vi "Example_Easy Save or Load Controls To From File.vi"() -> ()   [LabVIEW 2020]
doc: "Demonstrates how GUI object values can be saved into configuration file or loaded from the configuration file. This feature is extremely useful to manage settings of the application. Another, and very important, feature is that adding or removing items to be saved is taking minimum time."
uses:
  VI Server Toolkit LV2013.lvlib
  VI Server Libraries/VI Server Controls.llb/VI Server_GetSet Controls From String Format_Options.ctl
panel:
  in  "2D Array - Boolean":bool[][](array[boolean]) caption="2D Array - String"
  in  "2D Array - Path":path[][](array[path]) caption="2D Array - String"
  in  "EXIT":bool
  in  "LED":bool
  in  "Error In":errorcluster
  out "error out":errorcluster
  in  "SystemConfigurationFile":path caption="System Configuration File"
  in  "Load":bool
  in  "Save":bool
  in  "2D Array - String":string[][](array[string])
  in  "2D Array - DBL":dbl[][](array[numeric])
  in  "Menu Ring":u16(ring) items=["Item 1", "Item 2", "Item 3"]
  in  "1D Array - DBL":dbl[](array[numeric])
  in  "1D Array - String":string[](array[string])
  in  "Settings Button":bool
  in  "Knob":dbl(knob)=0.15380597915361302 scale=0.0..10.0
  in  "Horizontal Fill Slide":dbl(slide) scale=0.0..10.0
  in  "Numeric Control":dbl
  # "INSTRUCTIONS:\n\n1. Create the \"System configuration\" file path.\n2. Populate array elements, set controls and ring selection.\n3. Save the settings into configuration file (SAVE button).\n4. Change settings, empty arrays.\n5. Press LOAD button and verify the settings are properly updated.\n6. Examine the block diagram and note the Control Labels array which contains \nall labels of the saved/loaded controls."
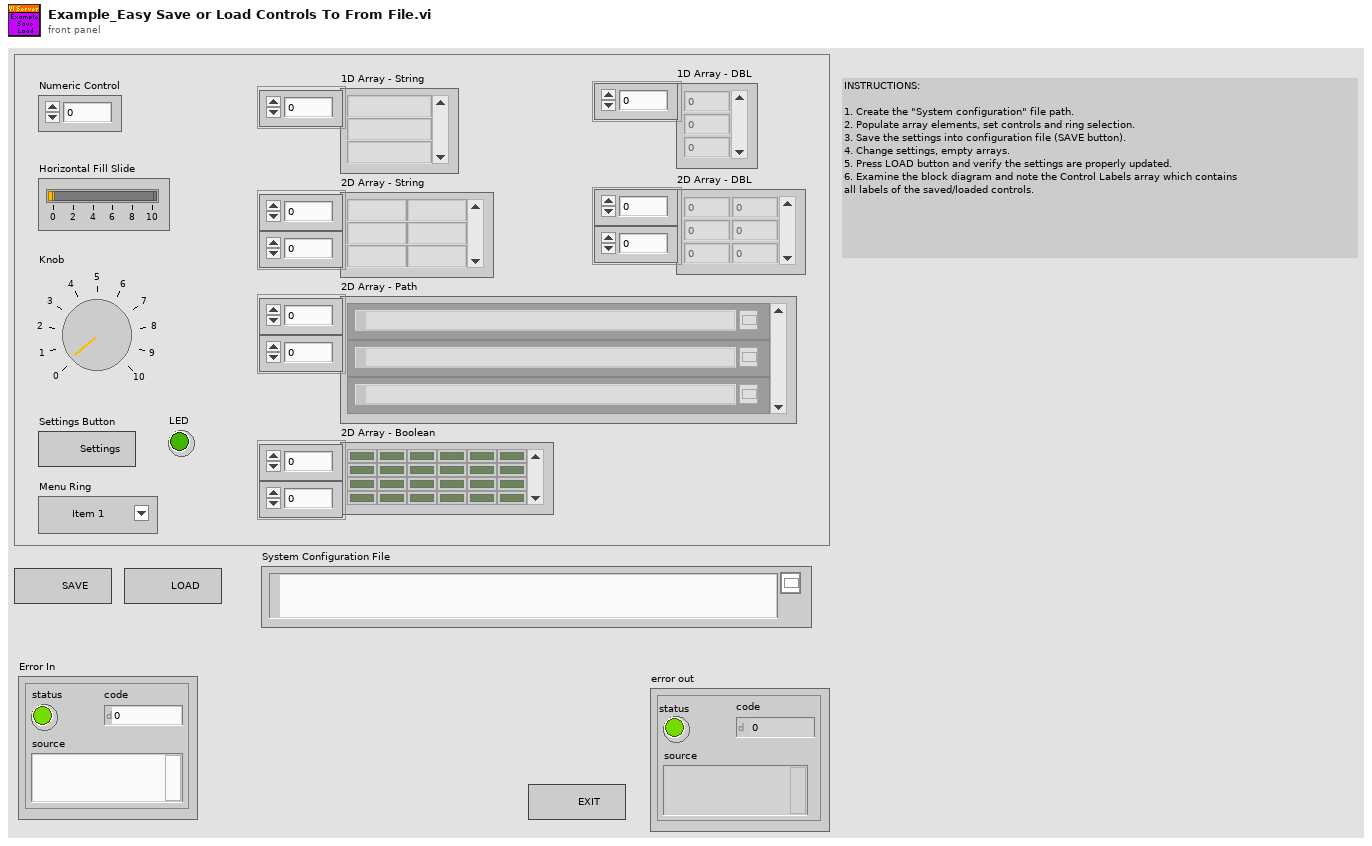
[diagram p1: front panel]
types:
  T1 = typedef "VI Server_RefsCluster.ctl" = cluster{"Labels":string[], "Refs":refnum<vi>[], "VI Ref":refnum<vi>}
  T2 = typedef "VI Server Toolkit LV2013.lvlib/VI Server_GetSet Controls From String Format_Options.ctl" = enum16{"", "If Ring Get Selection", "If Ring Set by Selection"}
  T3 = enum8{"Enabled", "Disabled", "Disabled and Grayed Out"}[]
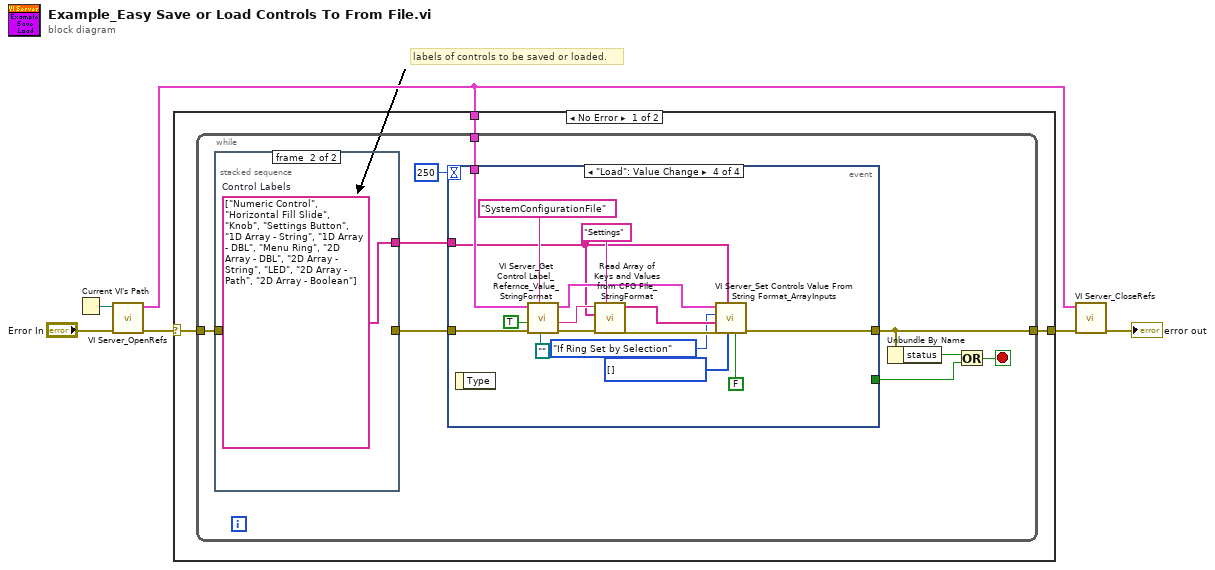
[diagram p0: block diagram]
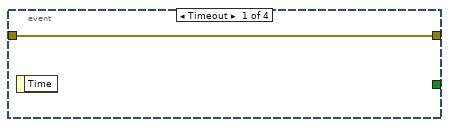
[diagram p2: hidden frame]
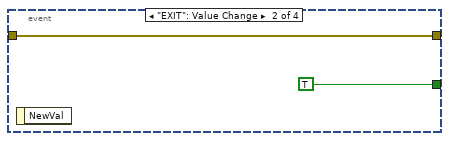
[diagram p3: hidden frame]
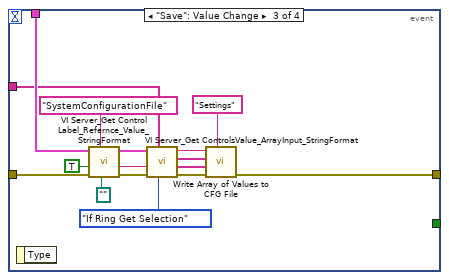
[diagram p4: hidden frame]
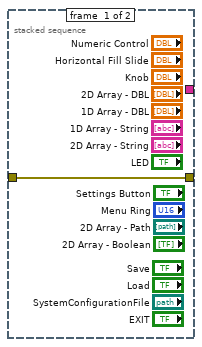
[diagram p5: hidden frame]
diagram:
  # "labels of controls to be saved or loaded."
  n1 = Current VI's Path() -> (path=w5:path)
  n2 = call "VI Server_OpenRefs.vi"("error in"="Error In", "VI Path"=w5) -> ("error out"=w4:errorcluster, "VI Server.RefsCluster"=w1:T1)  [unwired: 8 in]
  n3 = case shown="No Error" w4 {
    selector: w4 -> [w9 w55]
    tunnel: [w8 w55] -> w3
    tunnel: w1 -> [w7 _]
    frame No Error {
      n4 = while {
        tunnel: w9 -> [w17]
        tunnel: [w15] -> w8
        tunnel: w7 -> [w11]
        stop <- w12 stop-if-true
        n5 = stacked-sequence {
          tunnel: [w53 _] -> w16
          tunnel: w17 -> [w53 _]
          tunnel: [_ w54] -> w10
          frame #0 {
          }
          frame #1 {
            w54 = string[] ["Numeric Control", "Horizontal Fill Slide", "Knob", "Settings Button", "1D Array - String", "1D Array - DBL", "Menu Ring", "2D Array - DBL", "2D Array - String", "LED", "2D Array - Path", "2D Array - Boolean"]  # Control Labels
          }
        }
        n6 = event shown="[3] \"Load\": Value Change" {
          selector: _ -> [_ _ _ _]
          dyn-events: _ -> [_ _ _ _]
          timeout: 250 -> [_ _ _ _]
          tunnel: w16 -> [w19 w21 w33 w49]
          tunnel: [w19 w21 w22 w39] -> w15
          tunnel: [_ TRUE _ _] -> w13
          tunnel: w11 -> [_ _ w32 w48]
          tunnel: w10 -> [_ _ w28 w41]
          event Timeout {
            n7 = event-data() -> ()  [unwired: 1 in, 1 out]
          }
          event "EXIT": Value Change {
            n8 = event-data() -> ()  [unwired: 1 in, 1 out]
          }
          event "Save": Value Change {
            n9 = event-data() -> ()  [unwired: 1 in, 1 out]
            n10 = call "VI Server_Get Control Label_Refernce_Value_StringFormat.vi"(6:path "", "Label"="SystemConfigurationFile", "error in (no error)"=w33, 9:TRUE ("Single Instance (T)"), "VI Server Cluster"=w32) -> ("error out"=w31:errorcluster, "ControlValue(StringFormat)"=w26:string, "VI Server Cluster.DUP"=w30:T1)  [unwired: 4 in]
            n11 = call "VI Server_Get ControlsValue_ArrayInput_StringFormat.vi"("Options"=VI_Server_GetSet_Controls_From_String_Format_Options."If Ring Get Selection", "Labels.Array"=w28, "error in (no error)"=w31, "VI Server Cluster"=w30) -> ("error out"=w27:errorcluster, "Values.Array.STR"=w23:string[], "Labels.Array.DUP"=w24:string[])  [unwired: 3 in, 2 out]
            n12 = call "Write Array of Values to CFG File.vi"("Section"="Settings", "error in"=w27, "ValuesArray"=w23, "Keys Array"=w24, "CFG File Path"=w26) -> ("error out"=w22:errorcluster)  [unwired: 5 in, 1 out]
          }
          event "Load": Value Change {
            w38 = T3 [] items=["Enabled", "Disabled", "Disabled and Grayed Out"] ("Disabled")
            n13 = event-data() -> ()  [unwired: 1 in, 1 out]
            n14 = call "VI Server_Get Control Label_Refernce_Value_StringFormat.vi"(6:path "", "Label"="SystemConfigurationFile", "error in (no error)"=w49, 9:TRUE ("Single Instance (T)"), "VI Server Cluster"=w48) -> ("error out"=w47:errorcluster, "ControlValue(StringFormat)"=w46:string, "VI Server Cluster.DUP"=w42:T1)  [unwired: 4 in]
            n15 = call "Read Array of Keys and Values from CFG File_StringFormat.vi"("section"="Settings" ("Section"), "error in"=w47, "Keys Array"=w41, "GFG File Path"=w46) -> ("error out"=w44:errorcluster, "ValueArray (String)"=w43:string[])  [unwired: 6 in]
            n16 = call "VI Server_Set Controls Value From String Format_ArrayInputs.vi"("Value(Signaling. F=Value)"=FALSE, "Disabled"=w38, "Labels"=w41, "error in (no error)"=w44, "Values"=w43, "Options"=VI_Server_GetSet_Controls_From_String_Format_Options."If Ring Set by Selection", "VI Server Cluster"=w42) -> ("error out"=w39:errorcluster)  [unwired: 3 in, 1 out]
          }
        }
        n17 = Unbundle By Name(w15) -> ("status"=w14:bool)
        n18 = Or(x=w14, y=w13) -> (x .or. y?=w12:bool)
      }
    }
    frame Error {
    }
  }
  n19 = call "VI Server_CloseRefs.vi"("error in"=w3, "VI Server.RefsCluster"=w1) -> ("error out"=→"error out":errorcluster)  [unwired: 9 in]
